vi "TDS DCPS Set Voltage.vi"(8 "error in (no error)":errorcluster, 9 "Voltage":dbl, 10 "Signal InstConfig":string, 11 "Address":string) -> (0 "error out":errorcluster)   [LabVIEW 2025, in "Interface Functions.lvlib"]
uses:
  Interface Functions.lvlib
panel:
  out "VISA resource name out":refnum<visa-resource-name>
  # "DCPS Set Voltage"
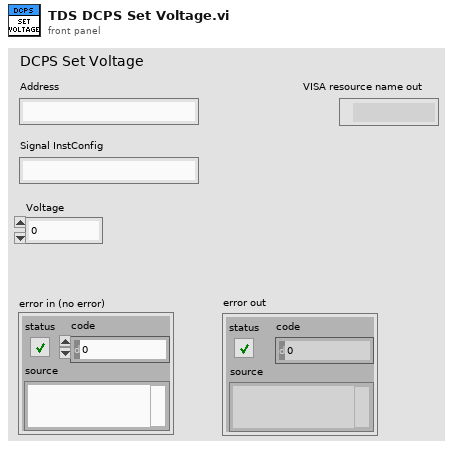
[diagram p1: front panel]
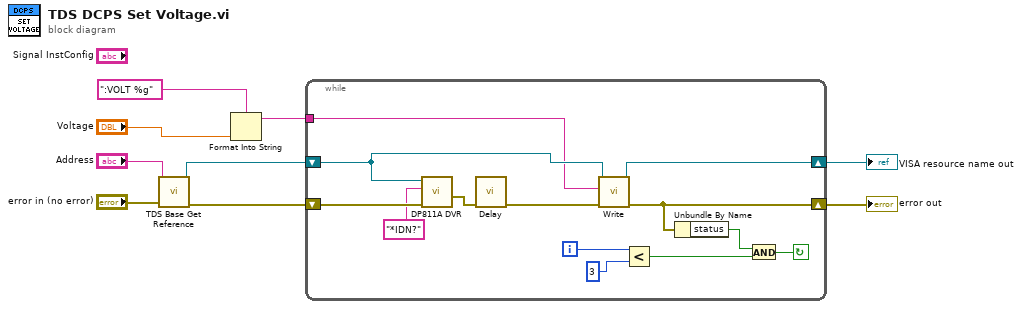
[diagram p0: block diagram]
diagram:
  n1 = call "TDS Base Get Reference.vi"("error in (no error)"="error in (no error)", "Address"="Address") -> ("error out"=w5:errorcluster, "Reference"=w3:refnum<visa-resource-name>)  [unwired: 8 in]
  n2 = Format Into String(format string=":VOLT %g", "Voltage") -> (resulting string=w2:string)  [unwired: 2 in, 1 out]
  n3 = while {
    tunnel: w2 -> [w12]
    shift-right: [w19] -> w4
    shift-left: w5 -> [w15]
    shift-right: [w22] -> w7
    shift-left: w3 -> [w13]
    i -> [w21]
    stop <- w16 continue-if-true
    n4 = call "DP811A DVR.vi"("error in (no error)"=w15, "write buffer"="*IDN?", "VISA resource name"=w13) -> ("error out"=w10:errorcluster)  [unwired: 3 in, 5 out]
    n5 = call "Delay"("error in (no error)"=w10) -> ("error out"=w14:errorcluster)  [unwired: 10 in]
    n6 = call "Write.vi"("error in (no error)"=w14, "Write Buffer (\"\")"=w12, "VISA resource name"=w13) -> ("error out"=w19:errorcluster, "VISA resource name out"=w22:refnum<visa-resource-name>)  [unwired: 7 in]
    n7 = Less?(x=w21, y=3) -> (x < y?=w17:bool)
    n8 = Unbundle By Name(w19) -> ("status"=w18:bool)
    n9 = And(x=w18, y=w17) -> (x .and. y?=w16:bool)
  }
  "error out" <- w4
  "VISA resource name out" <- w7
